vi "Send data by Email_2.vi"(3 "to":string="yehtingo@gmail.com", 4 "Attachment?":bool, 5 "plain text message":string="works?", 6 "Attachments path":path[](array[path]), 7 "subject":string="Test", 8 "error in":errorcluster, 9 "APP password":string="aiwfjsidudnfefes\n", 10 "username":string="ncuccc45002931", 11 "from":string="ncuccc45002931@gmail.com") -> (0 "error out":errorcluster)   [LabVIEW 2023]
uses:
  <vilib>/smtpClient/Set Message Text.vi
  <vilib>/smtpClient/LabVIEWSMTPClient.lvlib
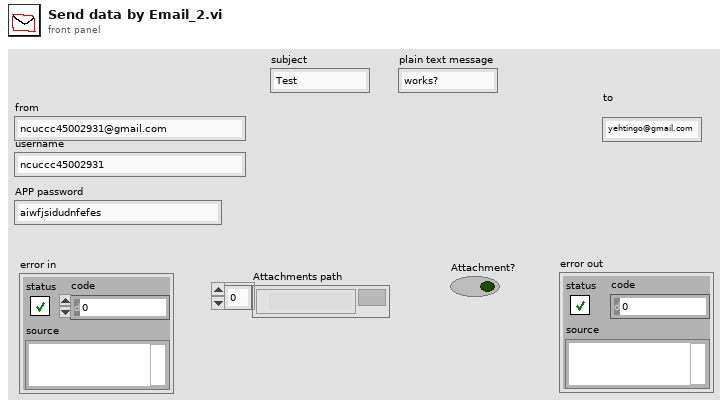
[diagram p1: front panel]
types:
  T1 = typedef "LabVIEWSMTPClient.lvlib/SmtpClientHandle.ctl" = refnum<k1>
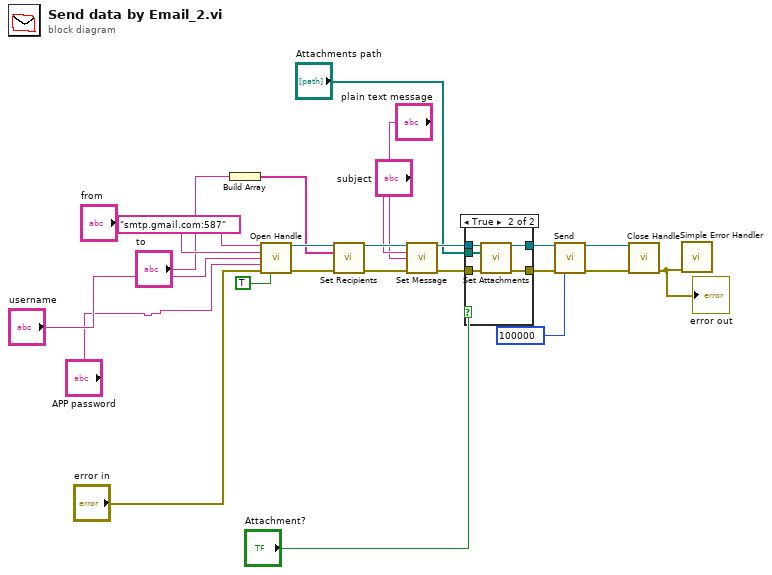
[diagram p0: block diagram]
diagram:
  n1 = Build Array("to") -> (w10:string[])
  n2 = call <vilib>:"Open Handle.vi"("server address"="smtp.gmail.com:587", "from"="from", "username"="username", "password"="APP password", "error in (no error)"="error in", "use TLS (false)"=TRUE) -> ("handle out"=w24:T1, "error out"=w23:errorcluster)  [unwired: 8 in]
  n3 = call <vilib>:"Set Recipients.vi"("handle in"=w24, "to"=w10, "error in (no error)"=w23) -> ("handle out"=w22:T1, "error out"=w21:errorcluster)  [unwired: 11 in]
  n4 = call-poly <vilib>:"Set Message.vi"("handle in"=w22, "subject"="subject", "plain text message"="plain text message", "error in (no error)"=w21) -> ("handle out"=w20:T1, "error out"=w19:errorcluster)  [unwired: 10 in]
  n5 = case shown="True" "Attachment?" {
    tunnel: w20 -> [w26 w31]
    tunnel: w19 -> [w25 w30]
    tunnel: [w26 w29] -> w18
    tunnel: [w25 w28] -> w17
    tunnel: "Attachments path" -> [_ w27]
    frame False {
    }
    frame True {
      n6 = call <vilib>:"Set Attachments.vi"("handle in"=w31, "attachments"=w27, "error in (no error)"=w30) -> ("handle out"=w29:T1, "error out"=w28:errorcluster)  [unwired: 11 in]
    }
  }
  n7 = call <vilib>:"Send.vi"("handle in"=w18, "error in (no error)"=w17, "timeout in ms (10000)"=100000) -> ("handle out"=w16:T1, "error out"=w15:errorcluster)  [unwired: 10 in, 1 out]
  n8 = call <vilib>:"Close Handle.vi"("handle in"=w16, "error in (no error)"=w15) -> ("error out"=w14:errorcluster)  [unwired: 12 in, 1 out]
  "error out" <- w14
  n9 = call <vilib>:"Simple Error Handler.vi"("error in (no error)"=w14) -> ()  [unwired: 4 in, 5 out]
